vi "FB_MFA_Read_Position_ENC.vi"() -> (3 "Position Get":sgl format="%.2f")   [LabVIEW 2011]
panel:
  out "error Position Get":errorcluster
  out "AAABuild":i32
  in  "MintController":refnum<k7>(container)
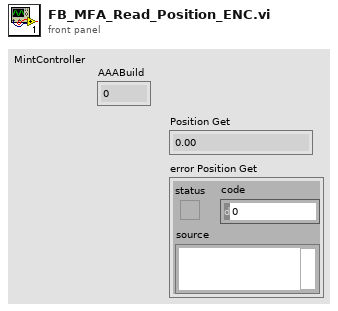
[diagram p1: front panel]
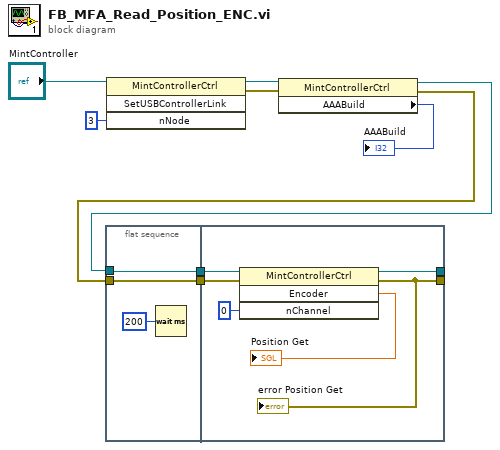
[diagram p0: block diagram]
diagram:
  n1 = flat-sequence {
    tunnel: w4 -> [w11]
    tunnel: [w11] -> w3
    tunnel: w2 -> [w10]
    tunnel: [w10] -> w1
    tunnel: [w16] -> _
    tunnel: [w15] -> _
    tunnel: w3 -> [w14]
    tunnel: w1 -> [w13]
    frame #0 {
      n2 = Wait (ms)(milliseconds to wait=u32 200) -> ()  [unwired: 1 out]
    }
    frame #1 {
      n3 = invoke class="MintControllerCtrl" method="Encoder"(reference=w14, error in=w13, "nChannel"=i16 0 ("nBank")) -> (reference out=w16:refnum<k7>, error out=w15:errorcluster, "Encoder"=→"Position Get":sgl)  [unwired: 1 in, 1 out]
      "error Position Get" <- w15
    }
  }
  n4 = invoke class="MintControllerCtrl" method="SetUSBControllerLink"(reference="MintController", "nNode"=i16 3 ("nNodeNumber")) -> (reference out=w9:refnum<k7>, error out=w6:errorcluster)  [unwired: 2 in, 2 out]
  n5 = property class="MintControllerCtrl"(reference=w9, error in=w6) -> (reference out=w4:refnum<k7>, error out=w2:errorcluster, "AAABuild"=→"AAABuild":i32)
